vi "SI.vi"() -> ()   [LabVIEW 2014]
doc: "This is the main user interface of the Raman spectroscopy system."
uses:
  TypeDef/GalvoInput.ctl
  TypeDef/States.ctl
panel:
  in  "Tab Control":enum32{"Main", "Galvo"}(tab)
  in  "Galvo Center":bool
  out "Galvo":bool
  in  "Quit":bool
  out "Initialization finished":bool
  in  "Galvo Stop":bool
  in  "Galvo Scan":bool
  out "CurrentFrame":i32
  in  "Scan parameters":T1={"area/um"=46.0417, "range_x/v"=0.6347, "range_y/v"=0.7773, "interval/um"=0.1806, "x_center/v"=3.35, "y_center/v"=5.55, "theta_1"=0.0, "theta_2"=60.0, "theta_3"=120.0}
  in  "Dir":i32=1
  in  "Phase":i32=1
  in  "delay/ms":u32=100
  in  "YOffset":dbl=5.55 caption="Offset"
  in  "XOffset":dbl=3.35 caption="Offset"
  out "Sample Rate":dbl=1000.0 format="%0.2f"
  out "Waveform Graph":waveform(dbl)[](graph)=[{"t0"=timestamp(0 s since 1904-01-01), "dt"=0.001, "Y"=[]}]
  in  "ZOffset":dbl=1.05 caption="Offset"
  in  "Galvo":T2={"Sample Rate"=2000000.0, "Sample Clock Source"="OnboardClock", "Max Voltage"=10.0, "Min Voltage"=-10.0, "Physical Channel(s)"="Dev1/ao0,Dev1/ao1,Dev1/ao3"}
  # "Objective: CFI Plan Fluor ELWD 60x (1.27 NA) \nThe depth of field: 1.78 um\nPixel Size: 0.0877um/px"
  # "Galvo Control"
  # "10^4>1s"
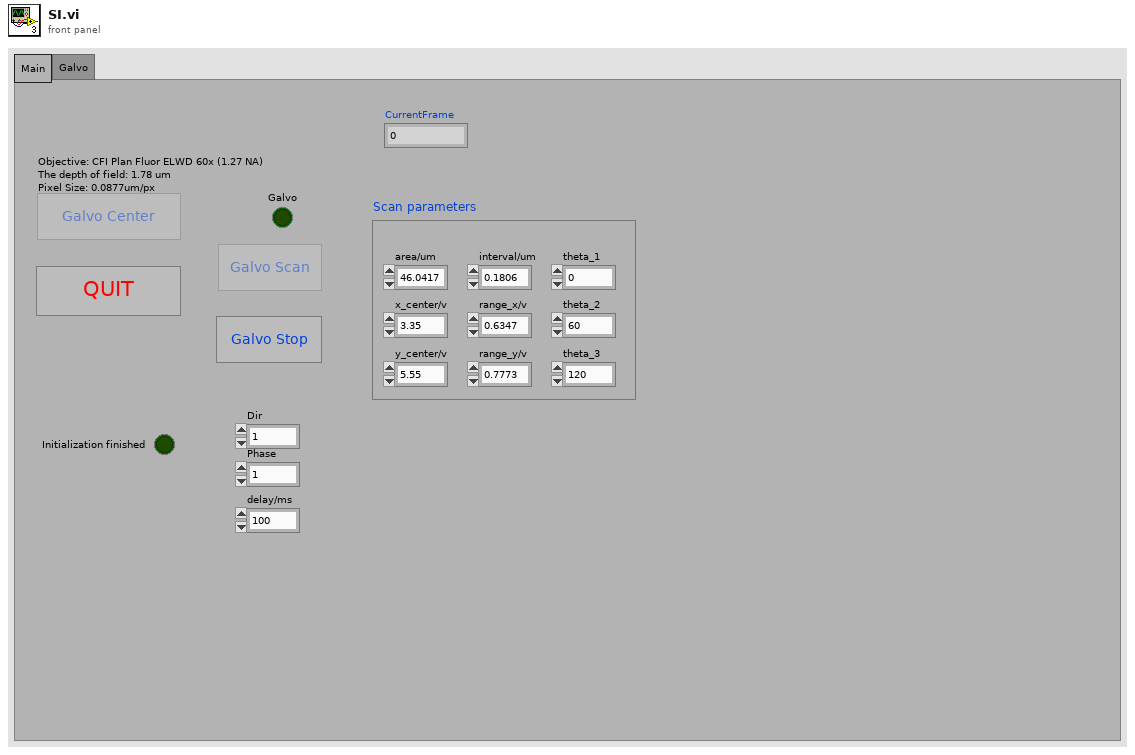
[diagram p1: front panel]
types:
  T1 = cluster{"area/um":dbl, "range_x/v":dbl, "range_y/v":dbl, "interval/um":dbl, "x_center/v":dbl, "y_center/v":dbl, "theta_1":dbl, "theta_2":dbl, "theta_3":dbl}
  T2 = typedef "GalvoInput.ctl" = cluster{"Sample Rate":dbl, "Sample Clock Source":tag, "Max Voltage":dbl, "Min Voltage":dbl, "Physical Channel(s)":tag}
  T3 = typedef "States.ctl" = enum16{"Initialize", "CMOS live", "Shut down"}
  T4 = enum8{"Enabled", "Disabled", "Disabled and Grayed Out"}
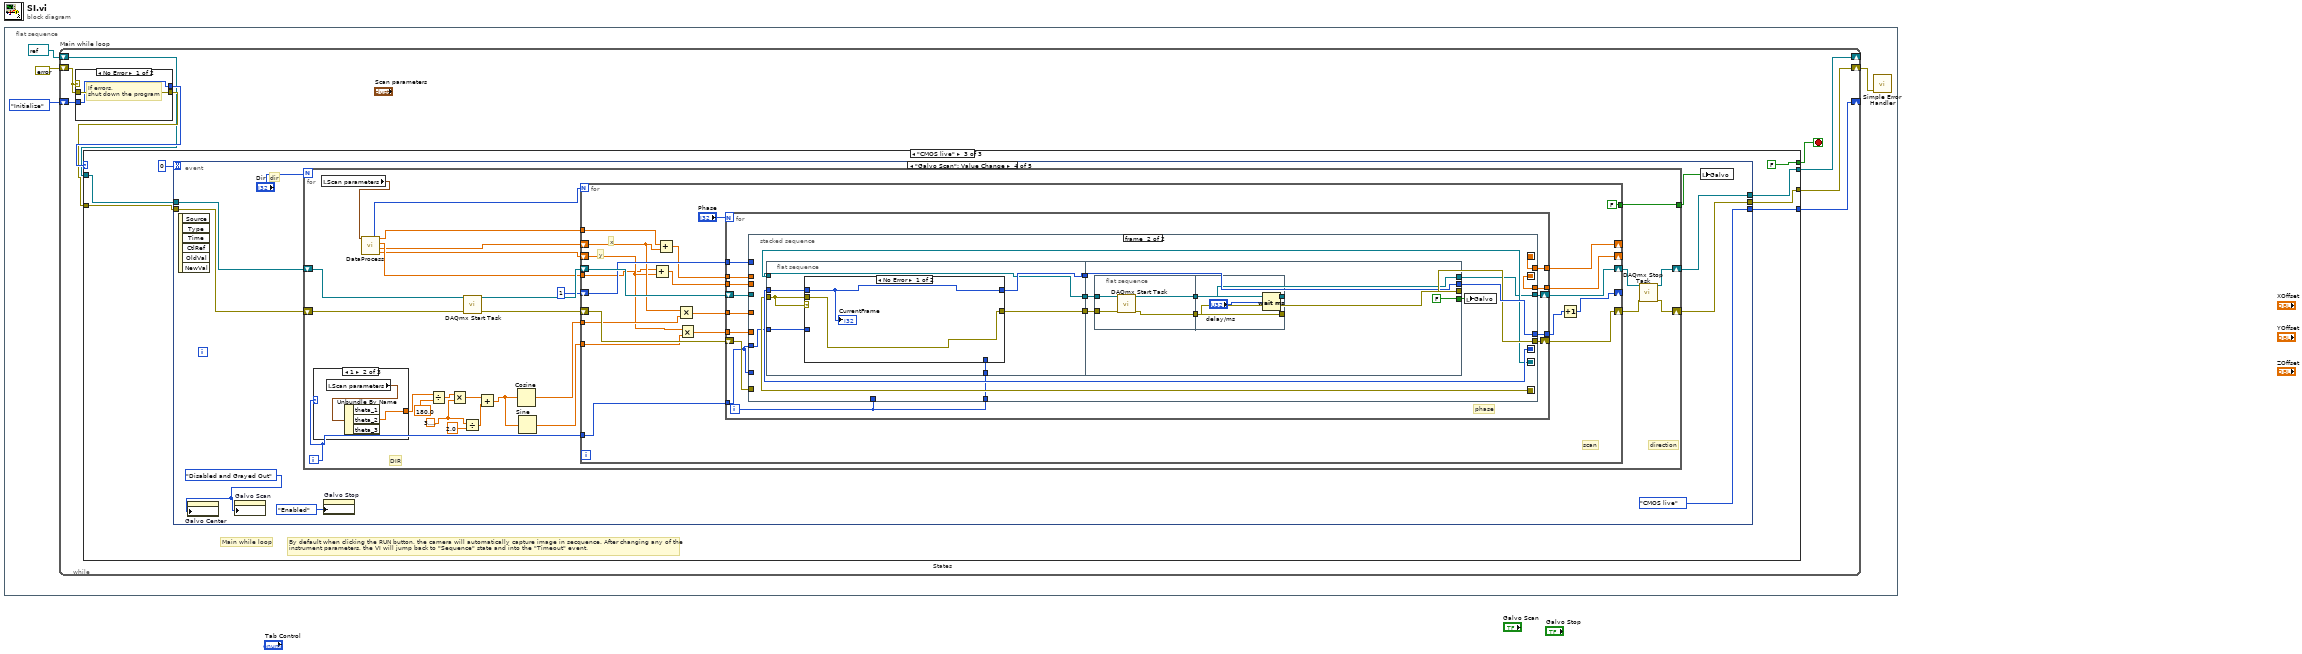
[diagram p0: block diagram]
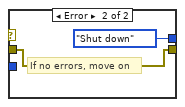
[diagram p2: hidden frame]
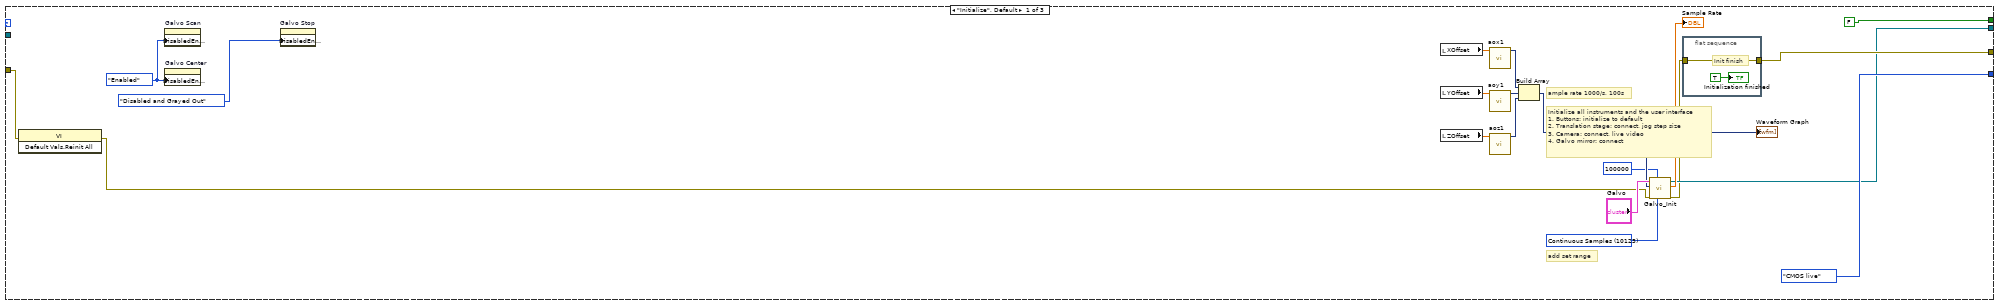
[diagram p3: hidden frame]
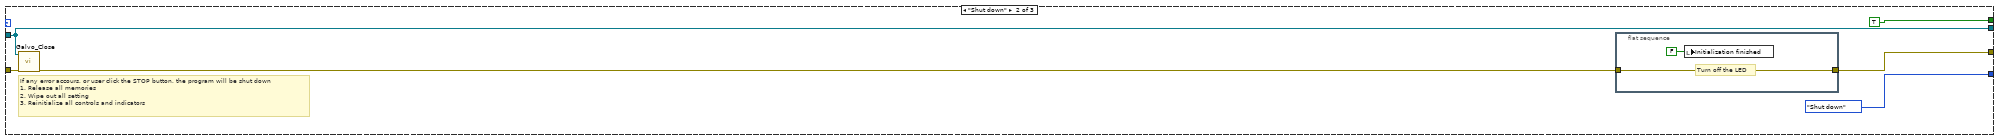
[diagram p4: hidden frame]
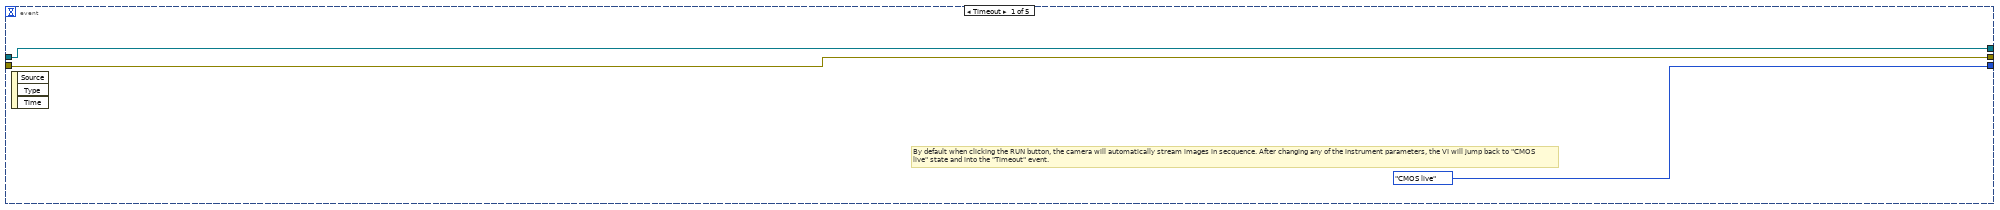
[diagram p5: hidden frame]
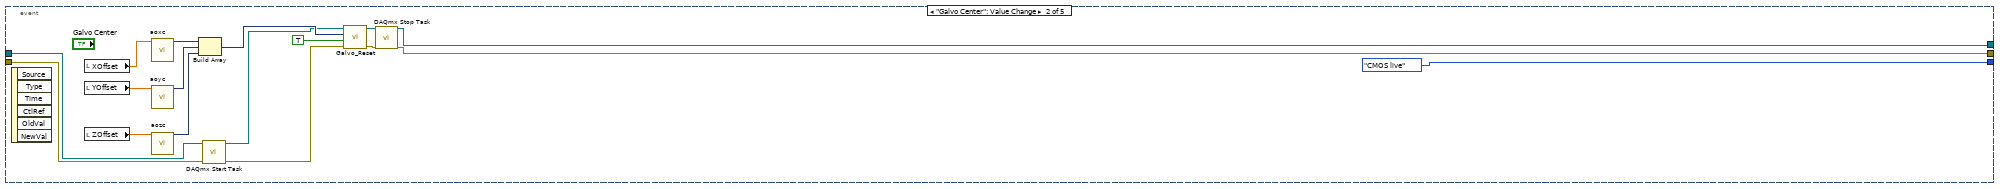
[diagram p6: hidden frame]
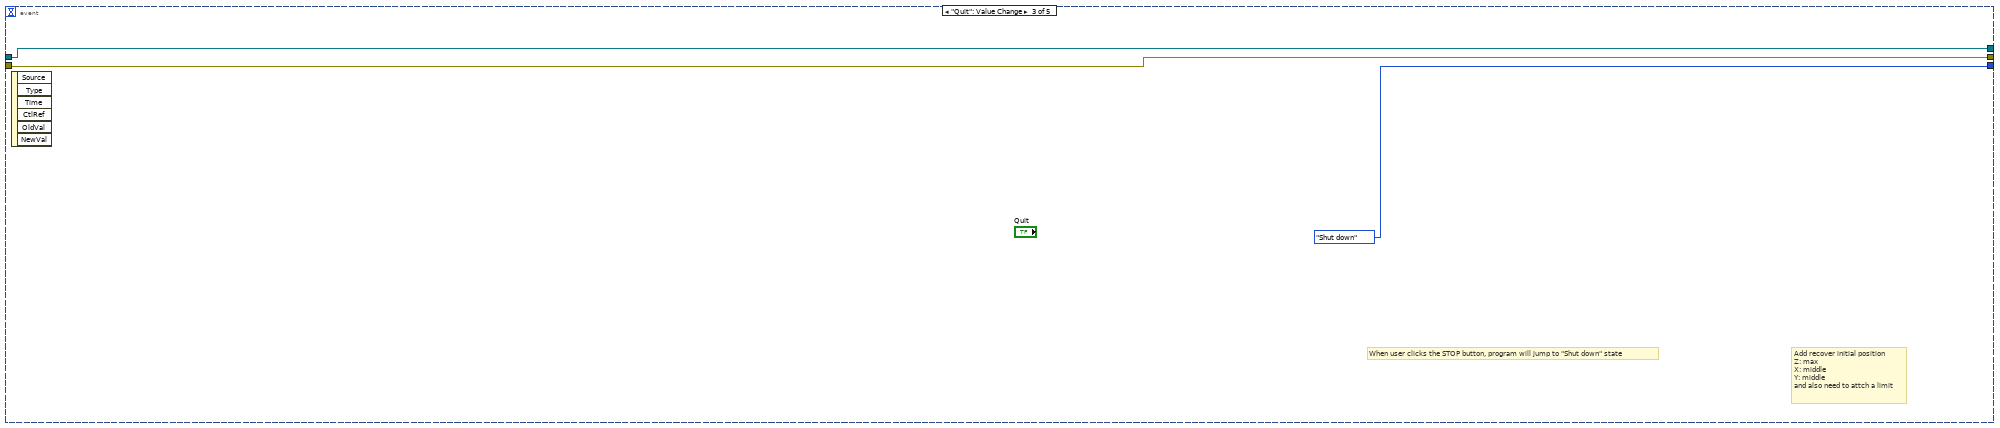
[diagram p7: hidden frame]
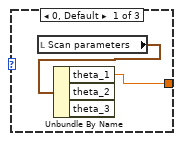
[diagram p8: hidden frame]
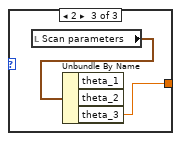
[diagram p9: hidden frame]
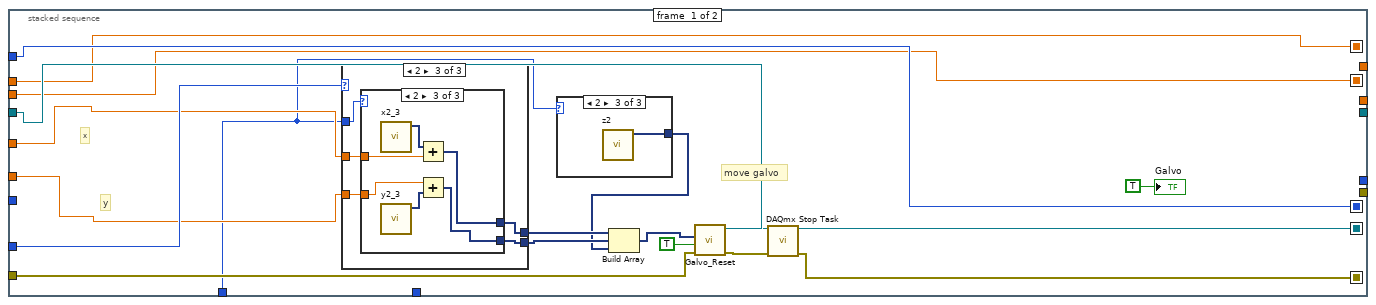
[diagram p10: hidden frame]
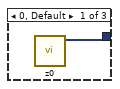
[diagram p11: hidden frame]
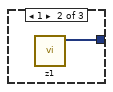
[diagram p12: hidden frame]
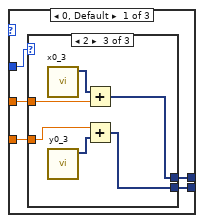
[diagram p13: hidden frame]
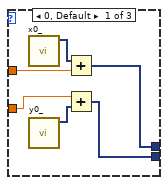
[diagram p14: hidden frame]
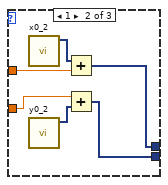
[diagram p15: hidden frame]
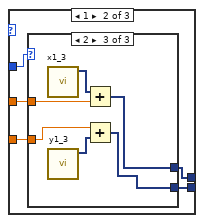
[diagram p16: hidden frame]
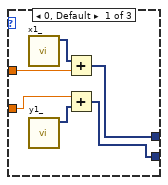
[diagram p17: hidden frame]
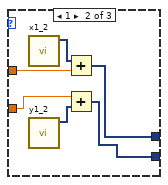
[diagram p18: hidden frame]
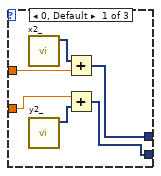
[diagram p19: hidden frame]
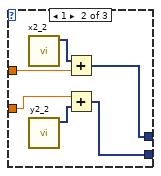
[diagram p20: hidden frame]
diagram:
  n1 = flat-sequence {
    frame #0 {
      n2 = while "Main while loop" {
        shift-right: [w8] -> _
        shift-left: States."Initialize" -> [w13]
        shift-right: [w11] -> w2
        shift-left: errorcluster {"status"=FALSE, "code"=0, "source"=""} ("error out") -> [w7]
        shift-right: [w6] -> _
        shift-left: refnum<k21> refnum ("task out") -> [w5]
        stop <- w9 stop-if-true
        n3 = case shown="No Error" w7 {
          tunnel: w7 -> [w15 w17]
          tunnel: [w15 w17] -> w10
          tunnel: w13 -> [w14 _]
          tunnel: [w14 States."Shut down"] -> w12
          frame No Error {
            # "If errors,\nshut down the program"
          }
          frame Error {
            # "If no errors, move on"
          }
        }
        n4 = case "States" shown="\"CMOS live\"" w12 {
          tunnel: [w35 w40 w52] -> w11
          tunnel: w10 -> [w36 w41 w53]
          tunnel: [FALSE TRUE FALSE] -> w9
          tunnel: [States."CMOS live" States."Shut down" w54] -> w8
          tunnel: [w32 w43 w49] -> w6
          tunnel: w5 -> [_ w43 w50]
          frame "Initialize", Default {
            w21 = T4."Enabled" ("Disabled")
            w27 = 10123 items=["Finite Samples"=10178, "Continuous Samples"=10123, "Hardware Timed Single Point"=12522] ("Sample Mode")
            # "ample rate 1000/s, 100s"
            # "add set range"
            # "Initialize all instruments and the user interface\n1. Buttons: initialize to default\n2. Translation stage: connect, jog step size\n3. Camera: connect, live video\n4. Galvo mirror: connect"
            n5 = invoke class="VI" method="Default Vals.Reinit All"(error in=w36) -> (error out=w20:errorcluster)  [unwired: 2 in, 2 out]
            n6 = property on="Galvo Scan" class="Bool"("DisabledEnum"=w21) -> ()  [unwired: 2 in, 2 out]
            n7 = property on="Galvo Center" class="Bool"("DisabledEnum"=w21) -> ()  [unwired: 2 in, 2 out]
            n8 = property on="Galvo Stop" class="Bool"("DisabledEnum"=T4."Disabled and Grayed Out" ("Disabled")) -> ()  [unwired: 2 in, 2 out]
            n9 = local read "XOffset"() -> (w24:dbl)
            n10 = local read "YOffset"() -> (w23:dbl)
            n11 = local read "ZOffset"() -> (w22:dbl)
            n12 = call "aox1"("Offset"=w24) -> ("DC"=w26:dynamicdata)  [unwired: 13 in, 1 out]
            n13 = call "aoy1"("Offset"=w23) -> ("DC"=w25:dynamicdata)  [unwired: 13 in, 1 out]
            n14 = call "aoz1"("Offset"=w22) -> ("DC"=w30:dynamicdata)  [unwired: 13 in, 1 out]
            n15 = Build Array(w26, w25, w30) -> (w29:dynamicdata[])
            "Waveform Graph" <- w29
            n16 = call "Galvo_Init.vi"("Sample Mode"=w27, "samples per channel"=100000, "error in"=w20, "Signal array"=w29, "Galvo_Input"="Galvo") -> ("error out"=w31:errorcluster, "Actual Sample Rate"=→"Sample Rate":dbl, "task out"=w32:refnum<k21>)  [unwired: 4 in]
            n17 = flat-sequence {
              tunnel: w31 -> [w39]
              tunnel: [w39] -> w35
              frame #0 {
                # "Init finish"
                "Initialization finished" <- TRUE ("Initialization finished")
              }
            }
          }
          frame "Shut down" {
            # "If any error accours, or user click the STOP button, the program will be shut down\n1. Release all memories\n2. Wipe out all setting\n3. Reinitialize all controls and indicators"
            n18 = call "Galvo_Close.vi"("error in"=w41, "task/channels in"=w43) -> ("error out"=w42:errorcluster)  [unwired: 9 in]
            n19 = flat-sequence {
              tunnel: w42 -> [w46]
              tunnel: [w46] -> w40
              frame #0 {
                # "Turn off the LED"
                n20 = local write "Initialization finished"(FALSE ("Initialization finished")) -> ()
              }
            }
          }
          frame "CMOS live" {
            # "Main while loop"
            # "By default when clicking the RUN button, the camera will automatically capture image in secquence. After changing any of the \ninstrument parameters, the VI will jump back to \"Sequence\" state and into the \"Timeout\" event."
            n21 = event shown="[3] \"Galvo Scan\": Value Change" {
              selector: _ -> [_ _ _ _ _]
              dyn-events: _ -> [_ _ _ _ _]
              timeout: 0 -> [_ _ _ _ _]
              tunnel: [States."CMOS live" States."CMOS live" States."Shut down" States."CMOS live" States."CMOS live"] -> w54
              tunnel: w53 -> [w55 w66 w76 w84 w287]
              tunnel: [w55 w60 w76 w80 w287] -> w52
              tunnel: [w57 w61 w75 w79 w289] -> w49
              tunnel: w50 -> [w57 w68 w75 w85 w289]
              event Timeout {
                # "By default when clicking the RUN button, the camera will automatically stream images in secquence. After changing any of the instrument parameters, the VI will jump back to \"CMOS live\" state and into the \"Timeout\" event."
                n22 = event-data() -> ()  [unwired: 1 in, 3 out]
              }
              event "Galvo Center": Value Change {
                n23 = event-data() -> ()  [unwired: 1 in, 6 out]
                n24 = local read "XOffset"() -> (w59:dbl)
                n25 = local read "YOffset"() -> (w58:dbl)
                n26 = local read "ZOffset"() -> (w72:dbl)
                n27 = call "aoxc"("Offset"=w59) -> ("DC"=w70:dynamicdata)  [unwired: 13 in, 1 out]
                n28 = call "aoyc"("Offset"=w58) -> ("DC"=w69:dynamicdata)  [unwired: 13 in, 1 out]
                n29 = call "aozc"("Offset"=w72) -> ("DC"=w73:dynamicdata)  [unwired: 13 in, 1 out]
                n30 = Build Array(w70, w69, w73) -> (w71:dynamicdata[])
                n31 = call <vilib>:"DAQmx Start Task.vi"("task/channels in"=w68, "error in"=w66) -> ("task out"=w67:refnum<k21>, "error out"=w65:errorcluster)  [unwired: 12 in]
                n32 = call "Galvo_Reset.vi"("error in"=w65, "auto start"=TRUE, "Signal array"=w71, "task/channels in"=w67) -> ("error out"=w62:errorcluster, "task out"=w63:refnum<k21>)  [unwired: 6 in]
                n33 = call <vilib>:"DAQmx Stop Task.vi"("task/channels in"=w63, "error in"=w62) -> ("task out"=w61:refnum<k21>, "error out"=w60:errorcluster)  [unwired: 12 in]
              }
              event "Quit": Value Change {
                # "Add recover initial position\nZ: max\nX: middle\nY: middle\nand also need to attch a limit"
                # "When user clicks the STOP button, program will jump to \"Shut down\" state"
                n34 = event-data() -> ()  [unwired: 1 in, 6 out]
              }
              event "Galvo Scan": Value Change {
                w82 = T4."Disabled and Grayed Out" ("Disabled")
                # "dir"
                n35 = event-data() -> ()  [unwired: 1 in, 6 out]
                n36 = property on="Galvo Center" class="Bool"("DisabledEnum"=w82) -> ()  [unwired: 2 in, 2 out]
                n37 = property on="Galvo Scan" class="Bool"("DisabledEnum"=w82) -> ()  [unwired: 2 in, 2 out]
                n38 = for {
                  N: "Dir" -> [_]
                  tunnel: [w111] -> w81
                  shift-right: [w87] -> w79
                  shift-left: w85 -> [w113]
                  shift-right: [w88] -> w80
                  shift-left: w84 -> [w108]
                  i -> [w107]
                  w102 = 3.141592653589793
                  # "direction"
                  # "DIR"
                  n39 = case shown="1" w107 {
                    tunnel: [w114 w116 w118] -> w105
                    frame 0, Default {
                      n40 = local read "Scan parameters"() -> (w115:T1)
                      n41 = Unbundle By Name(w115) -> ("theta_1"=w114:dbl)  [unwired: 2 out]
                    }
                    frame 1 {
                      n42 = local read "Scan parameters"() -> (w117:T1)
                      n43 = Unbundle By Name(w117) -> ("theta_2"=w116:dbl)  [unwired: 2 out]
                    }
                    frame 2 {
                      n44 = local read "Scan parameters"() -> (w119:T1)
                      n45 = Unbundle By Name(w119) -> ("theta_3"=w118:dbl)  [unwired: 2 out]
                    }
                  }
                  n46 = local read "Scan parameters"() -> (w96:T1)
                  n47 = call "DataProcess.vi"("Scan parameters"=w96) -> ("ystart"=w91:dbl, "xstart"=w92:dbl, "ystep"=w93:dbl, "xstep"=w94:dbl, "NUM"=w95:i32)  [unwired: 6 in]
                  n48 = Divide(x=w105, y=180.0) -> (x/y=w103:dbl)
                  n49 = Multiply(x=w103, y=w102) -> (x*y=w100:dbl)
                  n50 = Divide(x=w102, y=2.0) -> (x/y=w101:dbl)
                  n51 = call <vilib>:"DAQmx Start Task.vi"("task/channels in"=w113, "error in"=w108) -> ("task out"=w110:refnum<k21>, "error out"=w112:errorcluster)  [unwired: 12 in]
                  n52 = Add(x=w100, y=w101) -> (x+y=w99:dbl)
                  n53 = Cosine(x=w99) -> (cos(x)=w98:dbl)
                  n54 = Sine(x=w99) -> (sin(x)=w97:dbl)
                  n55 = for {
                    N: w95 -> [_]
                    tunnel: [FALSE ("Galvo")] -> w111
                    shift-right: [w140] -> w89
                    shift-left: w112 -> [w139]
                    shift-right: [w136] -> _
                    shift-left: w92 -> [w124]
                    shift-right: [w137] -> w90
                    shift-left: w110 -> [w138]
                    shift-right: [w132] -> _
                    shift-left: 1 -> [w135]
                    shift-right: [w134] -> _
                    shift-left: w91 -> [w123]
                    tunnel: w107 -> [w131]
                    tunnel: w98 -> [w128]
                    tunnel: w97 -> [w127]
                    tunnel: w94 -> [w122]
                    tunnel: w93 -> [w121]
                    # "scan"
                    # "y"
                    # "x"
                    n56 = Add(x=w121, y=w123) -> (x+y=w129:dbl)
                    n57 = Add(x=w122, y=w124) -> (x+y=w130:dbl)
                    n58 = Multiply(x=w124, y=w128) -> (x*y=w126:dbl)
                    n59 = Multiply(x=w123, y=w127) -> (x*y=w125:dbl)
                    n60 = for {
                      N: "Phase" -> [_]
                      tunnel: w130 -> [w153]
                      tunnel: w129 -> [w152]
                      tunnel: [w148] -> w134
                      tunnel: [w147] -> w136
                      shift-right: [w149] -> w140
                      shift-left: w139 -> [w155]
                      shift-right: [w150] -> w137
                      shift-left: w138 -> [w154]
                      tunnel: w135 -> [w151]
                      tunnel: [w146] -> w133
                      tunnel: w131 -> [w145]
                      tunnel: w126 -> [w143]
                      tunnel: w125 -> [w142]
                      i -> [w144]
                      # "phase"
                      n61 = stacked-sequence {
                        seq-local: [w171 _] -> [_ w252]
                        seq-local: [w163 _] -> [_ w254]
                        seq-local: [w164 _] -> [_ w253]
                        seq-local: [w169 _] -> [_ w259]
                        seq-local: [w166 _] -> [_ w251]
                        tunnel: w155 -> [w173 _]
                        tunnel: w154 -> [w168 _]
                        tunnel: w153 -> [w164 _]
                        tunnel: w152 -> [w163 _]
                        tunnel: w151 -> [w169 _]
                        tunnel: [_ w254] -> w148
                        tunnel: [_ w253] -> w147
                        tunnel: [_ w257] -> w146
                        tunnel: [_ w256] -> w149
                        tunnel: [_ w249] -> w150
                        tunnel: w145 -> [_ w248]
                        tunnel: w144 -> [_ w247]
                        tunnel: w145 -> [w165 _]
                        tunnel: w144 -> [w160 _]
                        tunnel: w143 -> [w162 _]
                        tunnel: w142 -> [w161 _]
                        frame #0 {
                          # "y"
                          # "x"
                          # "move galvo"
                          n62 = case shown="2" w165 {
                            tunnel: w162 -> [w182 w205 w228]
                            tunnel: w161 -> [w181 w204 w227]
                            tunnel: w160 -> [w180 w203 w226]
                            tunnel: [w179 w202 w225] -> w159
                            tunnel: [w178 w201 w224] -> w158
                            frame 0, Default {
                              n63 = case shown="2" w180 {
                                tunnel: w182 -> [w186 w192 w198]
                                tunnel: w181 -> [w185 w191 w197]
                                tunnel: [w184 w190 w196] -> w179
                                tunnel: [w183 w189 w195] -> w178
                                frame 0, Default {
                                n64 = call "x0_"() -> ("Signal"=w188:dynamicdata)  [unwired: 9 in, 2 out]
                                n65 = call "y0_"() -> ("Signal"=w187:dynamicdata)  [unwired: 9 in, 2 out]
                                n66 = Add(x=w188, y=w186) -> (x+y=w184:dynamicdata)
                                n67 = Add(x=w185, y=w187) -> (x+y=w183:dynamicdata)
                                }
                                frame 1 {
                                n68 = call "x0_2"() -> ("Signal"=w194:dynamicdata)  [unwired: 9 in, 2 out]
                                n69 = call "y0_2"() -> ("Signal"=w193:dynamicdata)  [unwired: 9 in, 2 out]
                                n70 = Add(x=w194, y=w192) -> (x+y=w190:dynamicdata)
                                n71 = Add(x=w191, y=w193) -> (x+y=w189:dynamicdata)
                                }
                                frame 2 {
                                n72 = call "x0_3"() -> ("Signal"=w200:dynamicdata)  [unwired: 9 in, 2 out]
                                n73 = call "y0_3"() -> ("Signal"=w199:dynamicdata)  [unwired: 9 in, 2 out]
                                n74 = Add(x=w200, y=w198) -> (x+y=w196:dynamicdata)
                                n75 = Add(x=w197, y=w199) -> (x+y=w195:dynamicdata)
                                }
                              }
                            }
                            frame 1 {
                              n76 = case shown="2" w203 {
                                tunnel: w205 -> [w209 w215 w221]
                                tunnel: w204 -> [w208 w214 w220]
                                tunnel: [w207 w213 w219] -> w202
                                tunnel: [w206 w212 w218] -> w201
                                frame 0, Default {
                                n77 = call "x1_"() -> ("Signal"=w211:dynamicdata)  [unwired: 9 in, 2 out]
                                n78 = call "y1_"() -> ("Signal"=w210:dynamicdata)  [unwired: 9 in, 2 out]
                                n79 = Add(x=w211, y=w209) -> (x+y=w207:dynamicdata)
                                n80 = Add(x=w208, y=w210) -> (x+y=w206:dynamicdata)
                                }
                                frame 1 {
                                n81 = call "x1_2"() -> ("Signal"=w217:dynamicdata)  [unwired: 9 in, 2 out]
                                n82 = call "y1_2"() -> ("Signal"=w216:dynamicdata)  [unwired: 9 in, 2 out]
                                n83 = Add(x=w217, y=w215) -> (x+y=w213:dynamicdata)
                                n84 = Add(x=w214, y=w216) -> (x+y=w212:dynamicdata)
                                }
                                frame 2 {
                                n85 = call "x1_3"() -> ("Signal"=w223:dynamicdata)  [unwired: 9 in, 2 out]
                                n86 = call "y1_3"() -> ("Signal"=w222:dynamicdata)  [unwired: 9 in, 2 out]
                                n87 = Add(x=w223, y=w221) -> (x+y=w219:dynamicdata)
                                n88 = Add(x=w220, y=w222) -> (x+y=w218:dynamicdata)
                                }
                              }
                            }
                            frame 2 {
                              n89 = case shown="2" w226 {
                                tunnel: w228 -> [w232 w238 w244]
                                tunnel: w227 -> [w231 w237 w243]
                                tunnel: [w230 w236 w242] -> w225
                                tunnel: [w229 w235 w241] -> w224
                                frame 0, Default {
                                n90 = call "x2_"() -> ("Signal"=w234:dynamicdata)  [unwired: 9 in, 2 out]
                                n91 = call "y2_"() -> ("Signal"=w233:dynamicdata)  [unwired: 9 in, 2 out]
                                n92 = Add(x=w234, y=w232) -> (x+y=w230:dynamicdata)
                                n93 = Add(x=w231, y=w233) -> (x+y=w229:dynamicdata)
                                }
                                frame 1 {
                                n94 = call "x2_2"() -> ("Signal"=w240:dynamicdata)  [unwired: 9 in, 2 out]
                                n95 = call "y2_2"() -> ("Signal"=w239:dynamicdata)  [unwired: 9 in, 2 out]
                                n96 = Add(x=w240, y=w238) -> (x+y=w236:dynamicdata)
                                n97 = Add(x=w237, y=w239) -> (x+y=w235:dynamicdata)
                                }
                                frame 2 {
                                n98 = call "x2_3"() -> ("Signal"=w246:dynamicdata)  [unwired: 9 in, 2 out]
                                n99 = call "y2_3"() -> ("Signal"=w245:dynamicdata)  [unwired: 9 in, 2 out]
                                n100 = Add(x=w246, y=w244) -> (x+y=w242:dynamicdata)
                                n101 = Add(x=w243, y=w245) -> (x+y=w241:dynamicdata)
                                }
                              }
                            }
                          }
                          n102 = case shown="2" w160 {
                            tunnel: [w175 w176 w177] -> w157
                            frame 0, Default {
                              n103 = call "z0"() -> ("Signal"=w175:dynamicdata)  [unwired: 9 in, 2 out]
                            }
                            frame 1 {
                              n104 = call "z1"() -> ("Signal"=w176:dynamicdata)  [unwired: 9 in, 2 out]
                            }
                            frame 2 {
                              n105 = call "z2"() -> ("Signal"=w177:dynamicdata)  [unwired: 9 in, 2 out]
                            }
                          }
                          n106 = Build Array(w159, w158, w157) -> (w156:dynamicdata[])
                          n107 = call "Galvo_Reset.vi"("error in"=w173, "auto start"=TRUE, "Signal array"=w156, "task/channels in"=w168) -> ("error out"=w172:errorcluster, "task out"=w167:refnum<k21>)  [unwired: 6 in]
                          n108 = call <vilib>:"DAQmx Stop Task.vi"("task/channels in"=w167, "error in"=w172) -> ("task out"=w166:refnum<k21>, "error out"=w171:errorcluster)  [unwired: 12 in]
                          "Galvo" <- TRUE
                        }
                        frame #1 {
                          n109 = flat-sequence {
                            tunnel: [w267] -> w260
                            tunnel: w259 -> [w266]
                            tunnel: [w265] -> w258
                            tunnel: w252 -> [w264]
                            tunnel: w251 -> [w263]
                            tunnel: [w263] -> w250
                            tunnel: w248 -> [w262]
                            tunnel: w247 -> [w261]
                            tunnel: [w274] -> w256
                            tunnel: w260 -> [w278]
                            tunnel: w258 -> [w279]
                            tunnel: [w279] -> w257
                            tunnel: [FALSE ("Galvo")] -> w255
                            tunnel: w250 -> [w276]
                            tunnel: [w275] -> w249
                            frame #0 {
                              n110 = case shown="No Error" w264 {
                                tunnel: [w268 w270] -> w267
                                tunnel: [w269 w271] -> w265
                                tunnel: w266 -> [w269 w271]
                                tunnel: w264 -> [w268 w270]
                                tunnel: w262 -> [_ _]
                                tunnel: w261 -> [_ _]
                                frame No Error {
                                "CurrentFrame" <- w269
                                }
                                frame Error {
                                (unwired) FALSE ("SaveStatus")
                                }
                              }
                            }
                            frame #1 {
                              n111 = flat-sequence {
                                tunnel: w278 -> [w283]
                                tunnel: w276 -> [w281]
                                tunnel: [w280] -> w273
                                tunnel: [w282] -> w272
                                tunnel: [w285] -> w275
                                tunnel: [w286] -> w274
                                tunnel: w273 -> [w286]
                                tunnel: w272 -> [w285]
                                frame #0 {
                                n112 = call <vilib>:"DAQmx Start Task.vi"("task/channels in"=w281, "error in"=w283) -> ("task out"=w282:refnum<k21>, "error out"=w280:errorcluster)  [unwired: 12 in]
                                }
                                frame #1 {
                                n113 = Wait (ms)(milliseconds to wait="delay/ms") -> ()  [unwired: 1 out]
                                }
                              }
                            }
                          }
                          n114 = local write "Galvo"(w255) -> ()
                        }
                      }
                    }
                    n115 = Increment(x=w133) -> (x+1=w132:i32)
                  }
                  n116 = call <vilib>:"DAQmx Stop Task.vi"("task/channels in"=w90, "error in"=w89) -> ("task out"=w87:refnum<k21>, "error out"=w88:errorcluster)  [unwired: 12 in]
                }
                n117 = property on="Galvo Stop" class="Bool"("DisabledEnum"=T4."Enabled" ("Disabled")) -> ()  [unwired: 2 in, 2 out]
                n118 = local write "Galvo"(w81) -> ()
              }
              event "Galvo Stop": Value Change {
                (unwired) T4."Disabled and Grayed Out" ("Disabled")
                w288 = T4."Enabled" ("Disabled")
                n119 = event-data() -> ()  [unwired: 1 in, 6 out]
                n120 = property on="Galvo Scan" class="Bool"("DisabledEnum"=w288) -> ()  [unwired: 2 in, 2 out]
                n121 = property on="Galvo Center" class="Bool"("DisabledEnum"=w288) -> ()  [unwired: 2 in, 2 out]
              }
            }
          }
        }
      }
      n122 = call <vilib>:"Simple Error Handler.vi"("error in (no error)"=w2) -> ()  [unwired: 4 in, 5 out]
    }
  }
